vi "Execute.vi"(8 "error in (no error)":errorcluster, 10 "Context in":refnum<class "Context.lvclass">, 11 "Start Command in":refnum<class "Start Command.lvclass">) -> (0 "error out":errorcluster, 2 "Context out":refnum<class "Context.lvclass">, 3 "Start Command out":refnum<class "Start Command.lvclass">)   [LabVIEW 2016, in "Start Command.lvclass"]
uses:
  Start Command.lvclass
  Context/Context.lvclass
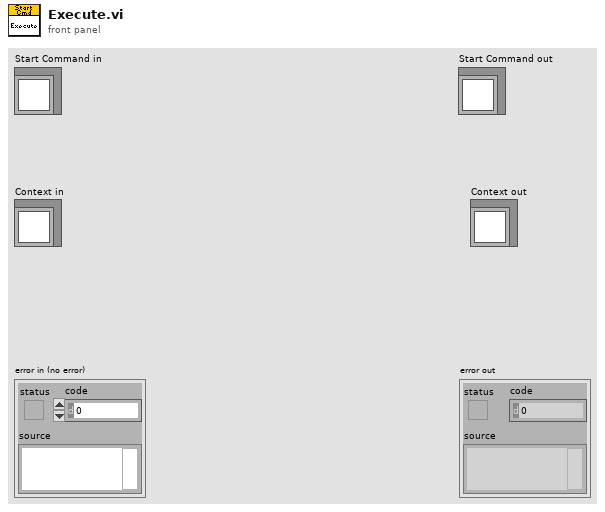
[diagram p1: front panel]
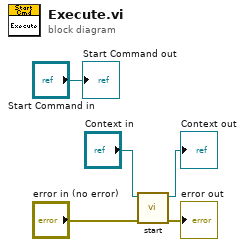
[diagram p0: block diagram]
diagram:
  n1 = call "start.vi"("error in (no error)"="error in (no error)", "Context in"="Context in") -> ("error out"=→"error out":errorcluster, "Context out"=→"Context out":refnum<class "Context.lvclass">)  [unwired: 8 in]
  "Start Command out" <- "Start Command in"
